vi "DIMPowerSupply.CheckVoltage.vi"(0 "i ref in":refnum<vi>, 3 "ms timeout (10000)":i32=10000, 5 "error in (no error)":errorcluster) -> (14 "i ref out":refnum<vi>, 17 "timed out":bool, 19 "error out":errorcluster)   [LabVIEW 2014, in "DIMPowerSupply.lvlib"]
doc: "Checks, if the actual voltage equals the nominal voltage by comparing the two values of the attribute data. The result is given as an indicator and published to DIM as well."
uses:
  DIMPowerSupply.lvlib
  CS_Core/CSApplicationBaseClasses/PSChannelBase/PSChannelBase.statusType.ctl
  CS_Core/CSApplicationBaseClasses/PSChannelBase/PSChannelBase.directionType.ctl
  CS_Core/CSApplicationBaseClasses/PSChannelBase/PSChannelBase.serviceType.ctl
  CS_Core/CSApplicationBaseClasses/PSChannelBase/PSChannelBase.lvlib
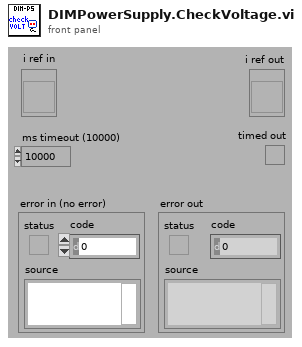
[diagram p1: front panel]
types:
  T1 = typedef "PSChannelBase.lvlib/PSChannelBase.serviceType.ctl" = enum16{"onOff", "voltage", "current", "tripCurrent", "rampUpSpeed", "rampDownSpeed", "status"}
  T2 = typedef "PSChannelBase.lvlib/PSChannelBase.directionType.ctl" = enum16{"unknown", "update actual value", "update nominal value", "update both"}
  T3 = typedef "PSChannelBase.lvlib/PSChannelBase.statusType.ctl" = i32
  T4 = typedef "DIMPowerSupply.lvlib/DIMPowerSupply.ranges type.ctl" = cluster{"deviceMin":dbl, "deviceMax":dbl, "numberMin":u16, "numberMax":u16, "U16?":bool, "factor":dbl}
  T5 = typedef "PSChannelBase.lvlib/PSChannelBase.i attribute.ctl" = cluster{"defaultChannelIndex":i32, "nofChannels":i32, "defaultChannelIndexID":i32, "nofChannelsID":i32, "actValues":T6, "nomValues":T6, "logicalName":string[], "physicalName":string[], "logicalNameID":i32, "physicalNameID":i32}
  T6 = typedef "PSChannelBase.lvlib/PSChannelBase.parameters.ctl" = cluster{"onOff":bool[], "voltage":dbl[], "current":dbl[], "tripCurrent":dbl[], "rampUpSpeed":dbl[], "rampDownSpeed":dbl[], "status":i32[], "serviceIDs":cluster{"onOfflID":i32, "voltageID":i32, "currentID":i32, "tripCurrentID":i32, "rampUpSpeedID":i32, "rampDownSpeedID":i32, "statusID":i32}}
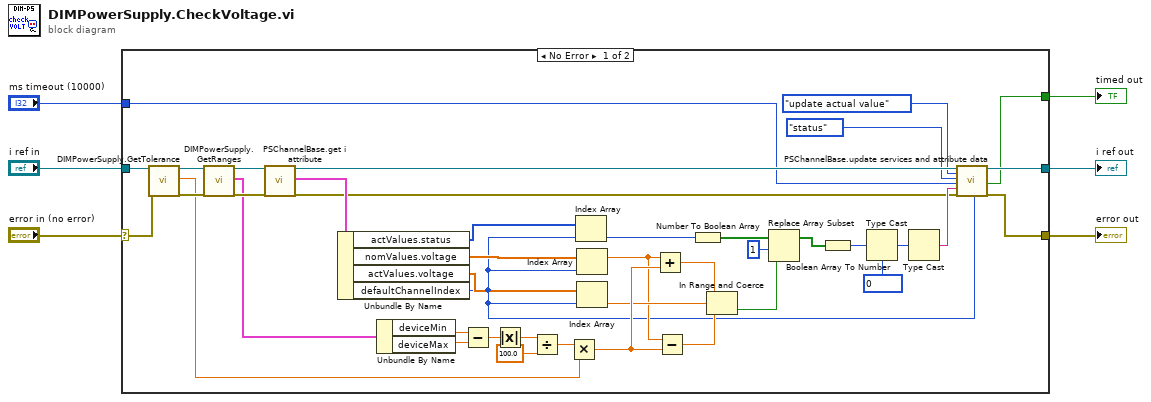
[diagram p0: block diagram]
diagram:
  n1 = case shown="No Error" "error in (no error)" {
    selector: "error in (no error)" -> [w46 w48]
    tunnel: "i ref in" -> [w45 w49]
    tunnel: "ms timeout (10000)" -> [w11 _]
    tunnel: [w9 w49] -> w4
    tunnel: [w8 w48] -> w3
    tunnel: [w7 _] -> w1
    frame No Error {
      w15 = T3 0 items=["onOff"=1, "inRange"=2, "rampingUp"=4, "rampingDown"=8, "tripped"=16, "error"=32] ("service")
      n2 = call "DIMPowerSupply.GetTolerance.vi"("i ref in"=w45, "error in (no error)"=w46) -> ("i ref out"=w44:refnum<vi>, "Tolerance"=w39:dbl, "error out"=w43:errorcluster)  [unwired: 15 in]
      n3 = call "DIMPowerSupply.GetRanges.vi"("i ref in"=w44, "error in (no error)"=w43) -> ("i ref out"=w42:refnum<vi>, "MonitorRanges"=w40:T4, "error out"=w41:errorcluster)  [unwired: 14 in, 1 out]
      n4 = call "PSChannelBase.get i attribute.vi"("i ref in"=w42, "error in (no error)"=w41) -> ("i ref out"=w19:refnum<vi>, "i attribute"=w47:T5, "error out"=w10:errorcluster)  [unwired: 15 in]
      n5 = Unbundle By Name(w47) -> ("actValues.status"=w20:i32[], "nomValues.voltage"=w27:dbl[], "actValues.voltage"=w38:dbl[], "defaultChannelIndex"=w16:i32)
      n6 = Unbundle By Name(w40) -> ("deviceMin"=w35:dbl, "deviceMax"=w36:dbl)
      n7 = Subtract(x=w35, y=w36) -> (x-y=w37:dbl)
      n8 = Absolute Value(x=w37) -> (abs(x)=w34:dbl)
      n9 = Divide(x=w34, y=100.0) -> (x/y=w32:dbl)
      n10 = Multiply(x=w32, y=w39) -> (x*y=w30:dbl)
      n11 = Index Array(array=w20, index=w16) -> (element=w25:i32)
      n12 = Index Array(array=w27, index=w16) -> (element=w26:dbl)
      n13 = Index Array(array=w38, index=w16) -> (element=w28:dbl)
      n14 = Add(x=w26, y=w30) -> (x+y=w31:dbl)
      n15 = Subtract(x=w26, y=w30) -> (x-y=w29:dbl)
      n16 = Number To Boolean Array(number=w25) -> (Boolean array=w24:bool[])
      n17 = In Range and Coerce(upper limit=w31, x=w28, lower limit=w29) -> (In Range?=w23:bool)  [unwired: 1 out]
      n18 = Replace Array Subset(array=w24, new element=w23, index=1) -> (w21:bool[])
      n19 = Boolean Array To Number(Boolean array=w21) -> (number=w14:u32)
      n20 = Type Cast(type=w15, x=w14) -> (*(type *) &x=w13:T3)
      n21 = Type Cast(x=w13) -> (*(type *) &x=w12:string)  [unwired: 1 in]
      n22 = call "PSChannelBase.update services and attribute data.vi"("i ref in"=w19, "direction"=PSChannelBase.directionType."update actual value", "service"=PSChannelBase.serviceType."status", "ms timeout (10000)"=w11, "value"=w12, "error in (no error)"=w10, "channelNumber"=w16) -> ("i ref out"=w9:refnum<vi>, "timed out"=w7:bool, "error out"=w8:errorcluster)  [unwired: 10 in]
    }
    frame Error {
    }
  }
  "error out" <- w3
  "i ref out" <- w4
  "timed out" <- w1
